vi "Stop Printing.vi"(8 "error in (no error)":errorcluster, 11 "Main.lvlib:Main.lvclass":refnum<class "Main.lvclass">) -> (0 "error out":errorcluster, 3 "Actor out":refnum<class "Actor.lvclass">)   [LabVIEW 2018, in "Main.lvlib" / "Main.lvclass"]
uses:
  Main.lvclass
  C:/Program Files/National Instruments/LabVIEW 2018/vi.lib/ActorFramework/Actor/Actor.lvclass
  <vilib>/ActorFramework/Actor/Actor.lvclass
  Main.lvclass/Main.ctl
  MFC Actor/MFC Messages/Change Setpoint Msg/Change Setpoint Msg.lvclass/Change Setpoint Msg.ctl
  <vilib>/ActorFramework/Message Enqueuer/Message Enqueuer.lvclass/Message Enqueuer.ctl
  <vilib>/ActorFramework/Message Enqueuer/Enqueue.vi
  MFC Actor/MFC Messages/Change Setpoint Msg/Change Setpoint Msg.lvclass
  C:/Program Files/National Instruments/LabVIEW 2018/vi.lib/ActorFramework/Message/Message.lvclass
  Feeder Actor/Feeder Messages/Stop Print Msg/Stop Print Msg.lvclass
  <vilib>/ActorFramework/Message Priority Queue/Priority Enqueue.vi
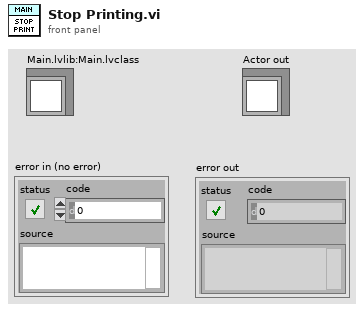
[diagram p1: front panel]
types:
  T1 = enum8{"Enabled", "Disabled", "Disabled and Grayed Out"}
  T2 = cluster{"Mixer Print Refnum":refnum<vi>, "Screw Print Refnum":refnum<vi>, "Inner Flow Print Refnum":refnum<vi>, "Outer Flow Print Refnum":refnum<vi>}
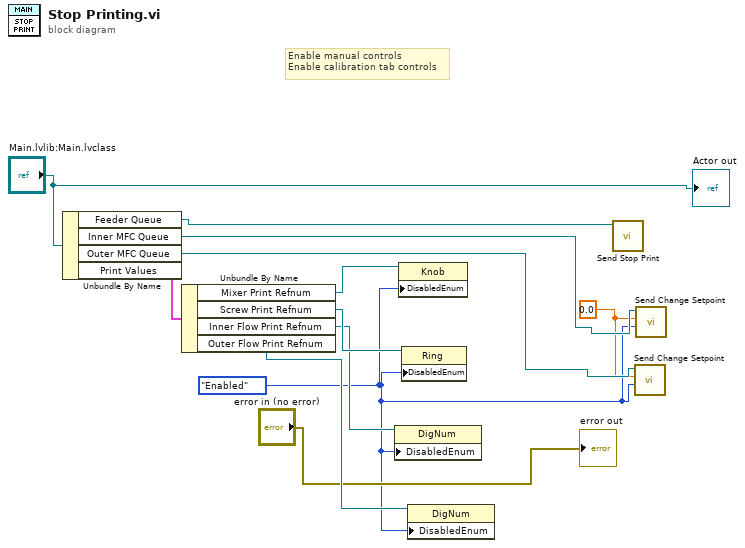
[diagram p0: block diagram]
diagram:
  w2 = 0.0 ("Setpoint")
  w1 = T1."Enabled" ("Disabled")
  # "Enable manual controls\nEnable calibration tab controls"
  n1 = Unbundle By Name("Main.lvlib:Main.lvclass") -> ("Feeder Queue"=w5:refnum<class "Message Enqueuer.lvclass">, "Inner MFC Queue"=w3:refnum<class "Message Enqueuer.lvclass">, "Outer MFC Queue"=w4:refnum<class "Message Enqueuer.lvclass">, "Print Values"=w12:T2)
  n2 = Unbundle By Name(w12) -> ("Mixer Print Refnum"=w11:refnum<vi>, "Screw Print Refnum"=w10:refnum<vi>, "Inner Flow Print Refnum"=w9:refnum<vi>, "Outer Flow Print Refnum"=w8:refnum<vi>)
  n3 = property class="DigNum"(reference=w9, "DisabledEnum"=w1) -> ()  [unwired: 1 in, 2 out]
  n4 = property class="Knob"(reference=w11, "DisabledEnum"=w1) -> ()  [unwired: 1 in, 2 out]
  n5 = property class="Ring"(reference=w10, "DisabledEnum"=w1) -> ()  [unwired: 1 in, 2 out]
  n6 = property class="DigNum"(reference=w8, "DisabledEnum"=w1) -> ()  [unwired: 1 in, 2 out]
  n7 = call "Send Stop Print.vi"("Message Enqueuer"=w5) -> ()  [unwired: 9 in, 2 out]
  n8 = call "Send Change Setpoint.vi"("Disabled"=w1, "Setpoint"=w2, "Message Enqueuer in"=w4) -> ()  [unwired: 7 in, 2 out]
  n9 = call "Send Change Setpoint.vi"("Disabled"=w1, "Setpoint"=w2, "Message Enqueuer in"=w3) -> ()  [unwired: 7 in, 2 out]
  "Actor out" <- "Main.lvlib:Main.lvclass"
  "error out" <- "error in (no error)"
